vi "PID % to EGU.vi"   [LabVIEW 2017, in "NI_PID_pid.lvlib"]
doc: "Converts percent of range input to engineering-units output based upon the min & max range settings. The output is normally limited to the range [max...min]. Values outside of the range [max..min] are allowed when the input coerce output to range? (T) is FALSE."
uses:
  <vilib>/addons/control/pid/NI_PID_pid.lvlib
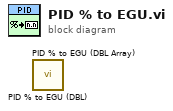
[diagram p0: block diagram]
diagram:
  n1 = call <vilib>:"PID % to EGU (DBL).vi"() -> ()  [unwired: 4 in, 1 out]
  n2 = call <vilib>:"PID % to EGU (DBL Array).vi"() -> ()  [unwired: 4 in, 1 out]
